vi "Handle Drop.vi"(4 "Mods":cluster{"Double Click":bool, "Menu Key":bool}, 5 "Tag":string, 6 "PlatMods":T2, 7 "Button":u16, 8 "error in (no error)":errorcluster, 9 "Coords":T1, 10 "Available Data Names":string[](array[string]), 11 "Test Executive View in":refnum<class "Test Executive View.lvclass">) -> (0 "error out":errorcluster, 2 "Discard?":bool, 3 "Test Executive View out":refnum<class "Test Executive View.lvclass">)   [LabVIEW 2017, in "Test Executive View.lvclass"]
uses:
  <vilib>/gpm_packages/@cs/Test-executive-builder/Example/Application/Test Executive View/Test Executive View/Test Executive View.lvclass
  C:/Program Files/National Instruments/LabVIEW 2017/vi.lib/gpm_packages/@cs/Test-executive-builder/Source/Test Executive Builder View/Test Executive Builder View/Test Executive Builder View.lvclass
  <vilib>/Utility/miscctls.llb/LVPoint32TypeDef.ctl
  <vilib>/gpm_packages/@cs/Test-executive-builder/Source/Test Executive Builder View/Test Executive Builder View/Test Executive Builder View.lvclass/Test Executive Builder View.ctl
  <vilib>/gpm_packages/@cs/Test-executive-builder/Source/Application Dependencies/Drop Element.ctl
  <vilib>/gpm_packages/@cs/Test-executive-builder/Source/Test Executive Builder View/Tree Click Interpreter/Tree Click Interpreter.lvclass
  <vilib>/gpm_packages/@cs/Test-executive-builder/Source/Test Executive Builder View/Test Executive Builder View/Test Executive Builder View.lvclass
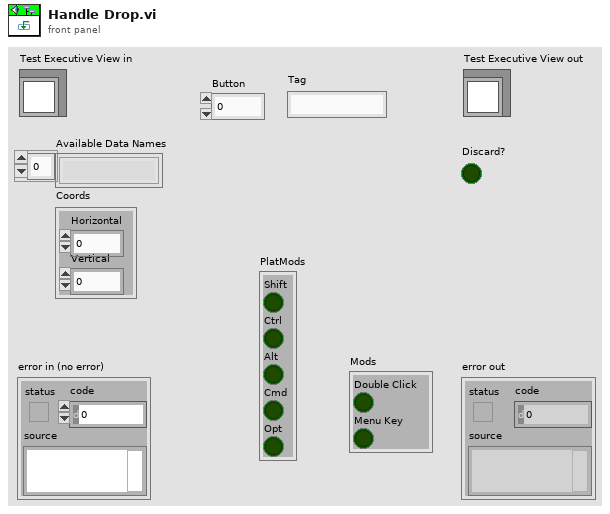
[diagram p1: front panel]
types:
  T1 = typedef "LVPoint32TypeDef.ctl" = cluster{"Horizontal":i32, "Vertical":i32}
  T2 = cluster{"Shift":bool, "Ctrl":bool, "Alt":bool, "Cmd":bool, "Opt":bool}
  T3 = typedef "Drop Element.ctl" = cluster{"Parent ID":string, "Insertion Index":i32, "Tag":string, "Ctrl":bool}
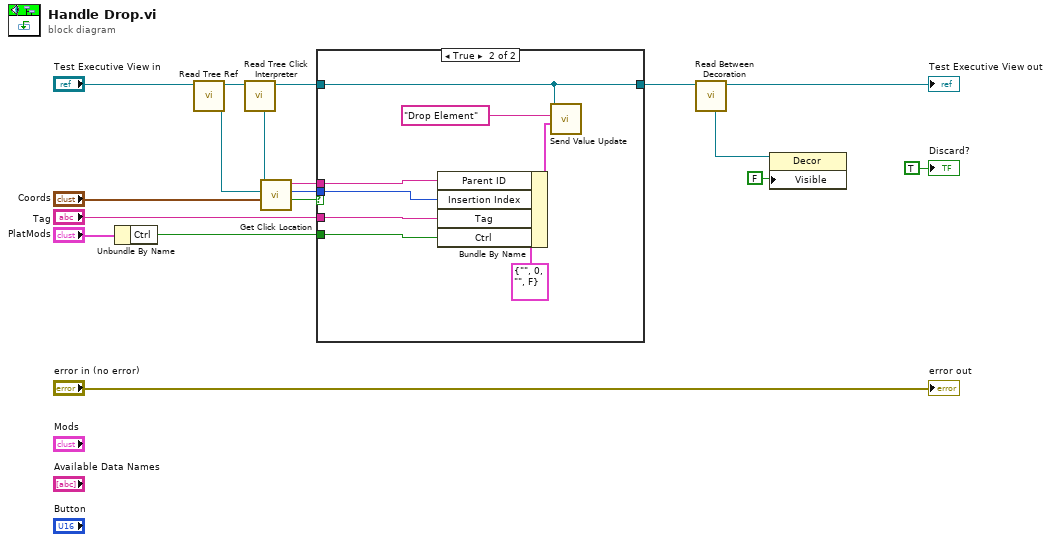
[diagram p0: block diagram]
diagram:
  n1 = Unbundle By Name("PlatMods") -> ("Ctrl"=w7:bool)
  n2 = call <vilib>:"Read Tree Ref.vi"("Test Executive Builder View in"="Test Executive View in") -> ("Tree Ref"=w12:refnum<vi>, "Test Executive Builder View out"=w16:refnum<class "Test Executive View.lvclass">)  [unwired: 9 in]
  n3 = call <vilib>:"Read Tree Click Interpreter.vi"("Test Executive Builder View in"=w16) -> ("Test Executive Builder View out"=w15:refnum<class "Test Executive View.lvclass">, "Tree Click Interpreter"=w13:refnum<class "Tree Click Interpreter.lvclass">)  [unwired: 9 in]
  n4 = call-dynamic "Get Click Location.vi"("Coords"="Coords", "Tree Refnum"=w12, "Tree Click Interpreter in"=w13) -> ("Valid?"=w5:bool, "Insertion Index"=w9:i32, "Parent ID"=w10:string)  [unwired: 4 in, 2 out]
  n5 = case shown="True" w5 {
    tunnel: w15 -> [w19 w21]
    tunnel: w10 -> [_ w25]
    tunnel: w9 -> [_ w24]
    tunnel: "Tag" -> [_ w23]
    tunnel: w7 -> [_ w22]
    tunnel: [w19 w21] -> w3
    frame False {
    }
    frame True {
      n6 = Bundle By Name(cluster=T3 {"Parent ID"="", "Insertion Index"=0, "Tag"="", "Ctrl"=FALSE} ("Drop Element"), "Parent ID"=w25, "Insertion Index"=w24, "Tag"=w23, "Ctrl"=w22) -> (w20:T3)
      n7 = call-dynamic "Send Value Update.vi"("Value"=w20, "Datum Name"="Drop Element", "IViewable in"=w21) -> ()  [unwired: 8 in, 1 out]
    }
  }
  n8 = call <vilib>:"Read Between Decoration.vi"("Test Executive Builder View in"=w3) -> ("Test Executive Builder View out"=→"Test Executive View out":refnum<class "Test Executive View.lvclass">, "Between Decoration"=w2:refnum<vi>)  [unwired: 9 in]
  n9 = property class="Decor"(reference=w2, "Visible"=FALSE) -> ()  [unwired: 1 in, 2 out]
  "error out" <- "error in (no error)"
  "Discard?" <- TRUE ("Discard?")
